vi "SubVI 2.vi"() -> ()   [LabVIEW 2011]
uses:
  ctlSeqFNs_SubVI 2.ctl
  ctlSeqFNs.ctl
  GLOBAL -MAIN.vi
panel:
  out "deg C":dbl[](array[numeric])
  out "deg F":dbl[](array[numeric])
  in  "STOP":bool
  out "Main Event Message":string
  # "Parellel SubVI 2"
  # "Receives data from SubVI 1 and converts Fahrenheit to Centigrade and sends to Main Program for plotting"
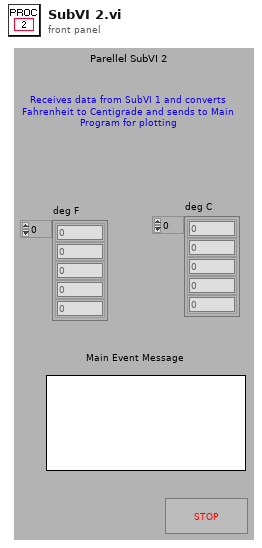
[diagram p1: front panel]
types:
  T1 = typedef "ctlSeqFNs_SubVI 2.ctl" = enum16{"INITIALIZE", "IDLE", "Convert deg F to deg C", "Send to Main", "Main Event Msg", "ERROR", "EXIT"}
  T2 = cluster{"VIRef":refnum<vi>, "Results":dbl[], "Queue Main":refnum<queue>}
  T3 = enum16{"ALIGN -CENTER", "ALIGN -TOP LEFT", "ALIGN -AS IS", "ALIGN -CUSTOM"}
  T4 = typedef "ctlSeqFNs.ctl" = enum16{"INITIALIZE MAIN", "INITIALIZE Sub", "IDLE", "Send Message to SubVIs", "PLOT RESULTS", "ERROR", "EXIT"}
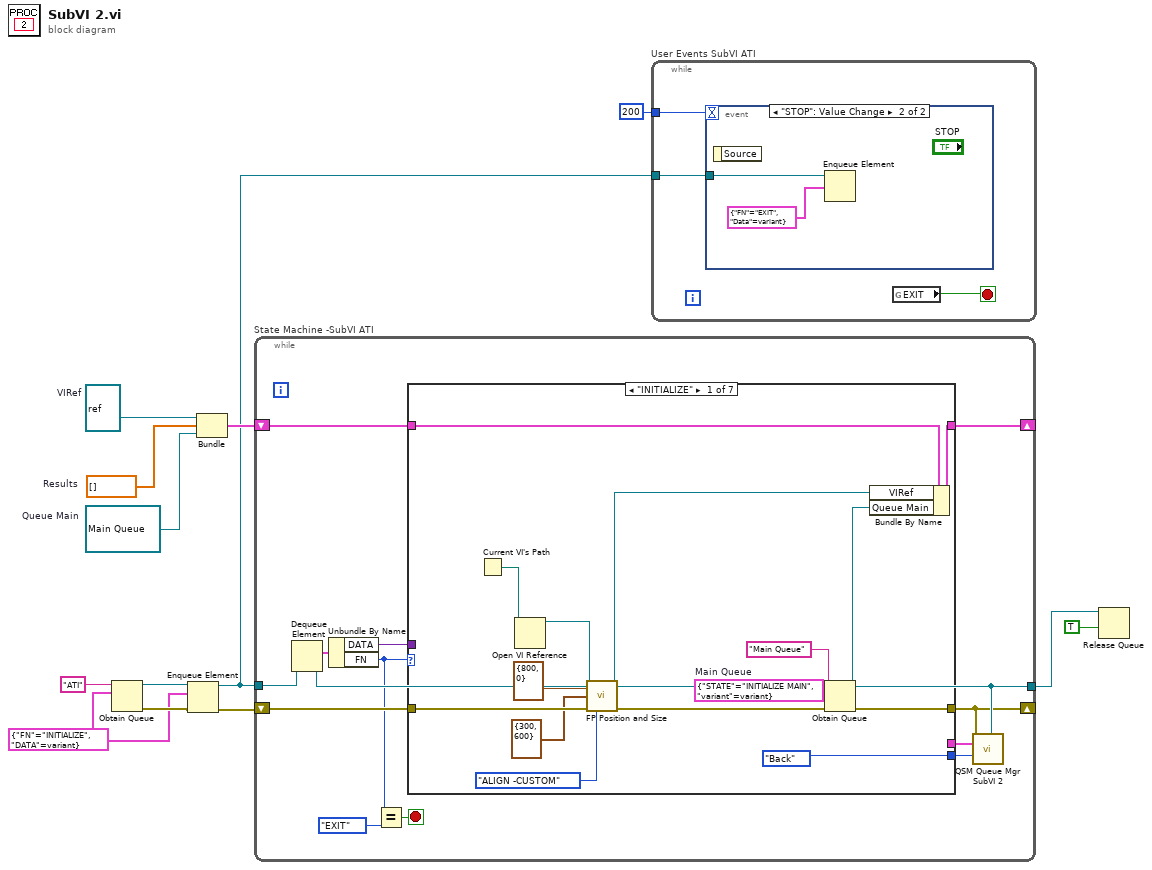
[diagram p0: block diagram]
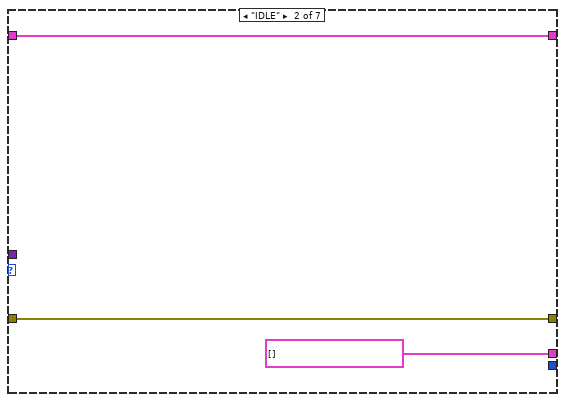
[diagram p2: hidden frame]
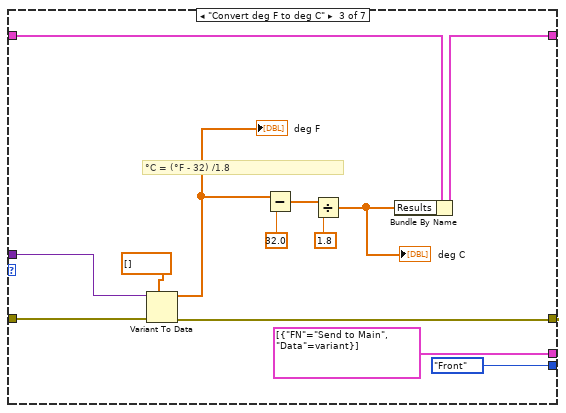
[diagram p3: hidden frame]
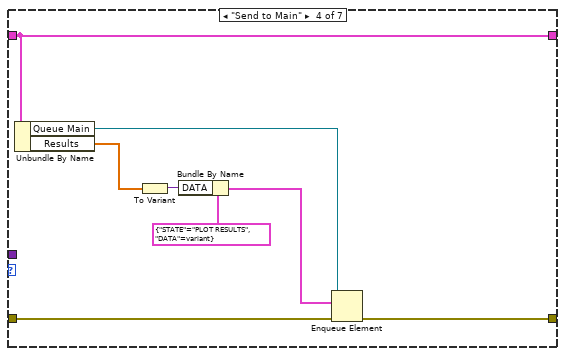
[diagram p4: hidden frame]
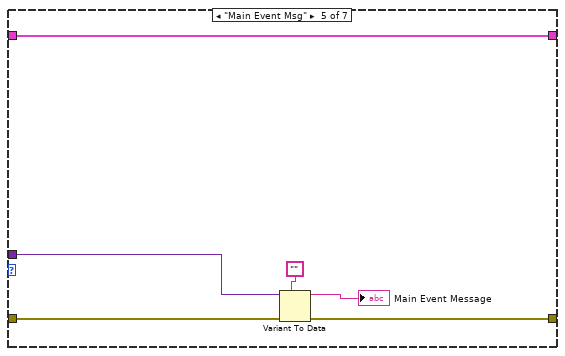
[diagram p5: hidden frame]
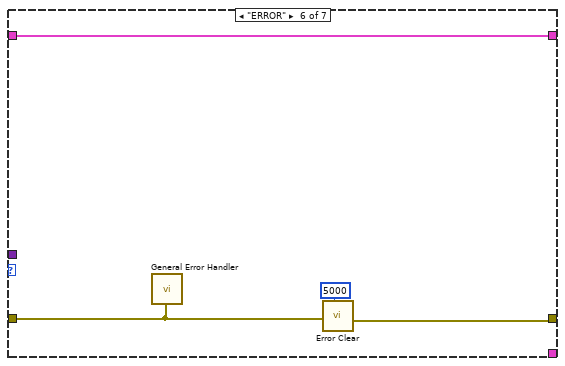
[diagram p6: hidden frame]
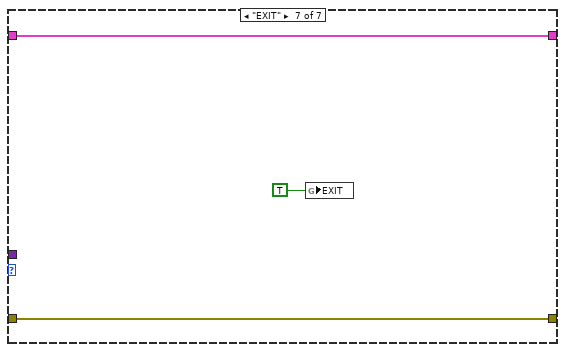
[diagram p7: hidden frame]
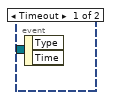
[diagram p8: hidden frame]
diagram:
  w2 = dbl[] []  # Results
  w3 = refnum<queue> refnum  # Queue Main
  w7 = refnum<vi> refnum  # VIRef
  w1 = cluster{"FN":T1, "DATA":variant} {"FN"=enum."INITIALIZE", "DATA"=variant} ("cluFNData")
  n1 = Obtain Queue(name (unnamed)="ATI", element data type=w1) -> (queue out=w9:refnum<queue>, error out=w11:errorcluster)  [unwired: 3 in, 1 out]
  n2 = Enqueue Element(queue=w9, element=w1, error in (no error)=w11) -> (queue out=w4:refnum<queue>, error out=w10:errorcluster)  [unwired: 1 in, 1 out]
  n3 = Bundle("VIRef"=w7, "Results"=w2, "Queue Main"=w3) -> (w8:T2)  [unwired: 1 in]
  n4 = while "State Machine -SubVI ATI" {
    shift-right: [w16] -> _
    shift-left: w10 -> [w26]
    tunnel: w4 -> [w23]
    tunnel: [w20] -> w6
    shift-right: [w17] -> _
    shift-left: w8 -> [w18]
    stop <- w25 stop-if-true
    n5 = Dequeue Element(queue=w23) -> (queue out=w20:refnum<queue>, element=w22:cluster{"FN":T1, "DATA":variant})  [unwired: 2 in, 2 out]
    n6 = Unbundle By Name(w22) -> ("DATA"=w21:variant, "FN"=w19:T1)
    n7 = Equal?(x=w19, y=ctlSeqFNs_SubVI_2."EXIT" ("FN")) -> (x = y?=w25:bool)
    n8 = case shown="\"INITIALIZE\"" w19 {
      tunnel: w26 -> [w37 w43 w57 w64 w67 w72 w77]
      tunnel: [w30 w43 w56 w63 w66 w74 w77] -> w16
      tunnel: w21 -> [_ _ w55 _ w70 _ _]
      tunnel: w18 -> [w36 w44 w48 w65 w71 w75 w78]
      tunnel: [w35 w44 w47 w65 w71 w75 w78] -> w17
      tunnel: [_ cluster{"FN":T1, "Data":variant}[] [] ("QFNs") cluster{"FN":T1, "Data":variant}[] [{"FN"=enum."Send to Main", "Data"=variant}] ("QFNs") _ _ _ _] -> w15
      tunnel: [enum16{"Back", "Front", "Replace"}."Back" ("Enum") _ enum16{"Back", "Front", "Replace"}."Front" ("Enum") _ _ _ _] -> w14
      frame "INITIALIZE" {
        w29 = cluster{"STATE":T4, "variant":variant} {"STATE"=enum."INITIALIZE MAIN", "variant"=variant}  # Main Queue
        n9 = Current VI's Path() -> (path=w40:path)
        n10 = Open VI Reference(vi path=w40) -> (vi reference=w39:refnum<vi>)  [unwired: 5 in, 1 out]
        n11 = call "FP Position and Size.vi"("VIRefNum  IN"=w39, "Poistion"=cluster{"left":i16, "top":i16} {"left"=800, "top"=0}, "Size"=cluster{"right":i16, "bottom":i16} {"right"=300, "bottom"=600}, "error in (no error)"=w37, "Mode"=T3."ALIGN -CUSTOM") -> ("VIRefNum OUT"=w38:refnum<vi>, "error out"=w31:errorcluster)  [unwired: 9 in]
        n12 = Obtain Queue(name (unnamed)="Main Queue", element data type=w29, error in (no error)=w31) -> (queue out=w27:refnum<queue>, error out=w30:errorcluster)  [unwired: 2 in, 1 out]
        n13 = Bundle By Name(cluster=w36, "VIRef"=w38, "Queue Main"=w27) -> (w35:T2)
      }
      frame "IDLE" {
      }
      frame "Convert deg F to deg C" {
        # "°C = (°F - 32) /1.8"
        n14 = Variant To Data(error in=w57, type=dbl[] [] ("deg F"), Variant=w55) -> (data=w45:dbl[], error out=w56:errorcluster)
        "deg F" <- w45
        n15 = Subtract(x=w45, y=32.0) -> (x-y=w52:dbl[])
        n16 = Divide(x=w52, y=1.8) -> (x/y=w46:dbl[])
        "deg C" <- w46
        n17 = Bundle By Name(cluster=w48, "Results"=w46) -> (w47:T2)
      }
      frame "Send to Main" {
        n18 = Unbundle By Name(w65) -> ("Queue Main"=w62:refnum<queue>, "Results"=w59:dbl[])
        n19 = To Variant(anything=w59) -> (Variant=w60:variant)
        n20 = Bundle By Name(cluster=cluster{"STATE":T4, "DATA":variant} {"STATE"=enum."PLOT RESULTS", "DATA"=variant} ("element"), "DATA"=w60) -> (w58:cluster{"STATE":T4, "DATA":variant})
        n21 = Enqueue Element(queue=w62, element=w58, error in (no error)=w64) -> (error out=w63:errorcluster)  [unwired: 1 in, 2 out]
      }
      frame "Main Event Msg" {
        n22 = Variant To Data(error in=w67, type="", Variant=w70) -> (data=→"Main Event Message":string, error out=w66:errorcluster)
      }
      frame "ERROR" {
        n23 = call <vilib>:"General Error Handler.vi"("error in (no error)"=w72) -> ()  [unwired: 10 in, 5 out]
        n24 = call "Error Clear.vi"("wait(ms)"=u32 5000, "error in"=w72) -> ("error in (no error)"=w74:errorcluster)  [unwired: 6 in]
      }
      frame "EXIT" {
        n25 = global write "GLOBAL -MAIN.vi" "EXIT"(TRUE ("EXIT")) -> ()
      }
    }
    n26 = call "QSM Queue Mgr SubVI 2.vi"("QSTATES"=w15, "QRef"=w20, "Error IN"=w16, "FNs"=w14) -> ()  [unwired: 11 in, 1 out]
  }
  n27 = while "User Events SubVI ATI" {
    tunnel: 200 -> [w81]
    tunnel: w4 -> [w79]
    stop <- w80 stop-if-true
    n28 = event shown="[1] \"STOP\": Value Change" {
      selector: _ -> [_ _]
      dyn-events: _ -> [_ _]
      timeout: w81 -> [_ _]
      tunnel: w79 -> [_ w83]
      event Timeout {
        n29 = event-data() -> ()  [unwired: 1 in, 2 out]
      }
      event "STOP": Value Change {
        n30 = event-data() -> ()  [unwired: 1 in, 1 out]
        n31 = Enqueue Element(queue=w83, element=cluster{"FN":T1, "Data":variant} {"FN"=enum."EXIT", "Data"=variant}) -> ()  [unwired: 2 in, 3 out]
      }
    }
    n32 = global read "GLOBAL -MAIN.vi" "EXIT"() -> (w80:bool)
  }
  n33 = Release Queue(queue=w6, force destroy? (F)=TRUE) -> ()  [unwired: 1 in, 3 out]
